vi "Replace Array Elements - string.vi"(4 "new elements (none)":string[](array[string])=["a"], 5 "indices (none)":i32[](array[numeric])=[3, 5], 7 "1D Array":string[](array[string])=["0", "1", "2", "empty", "4", "none", "6", "7", "8"]) -> (2 "output array":string[](array[string]))   [LabVIEW 2020]
doc: "Replaces elements in a 1-dim array at the specified indices. This is a list-based version of the built-in \"Replace Array Subset\"."
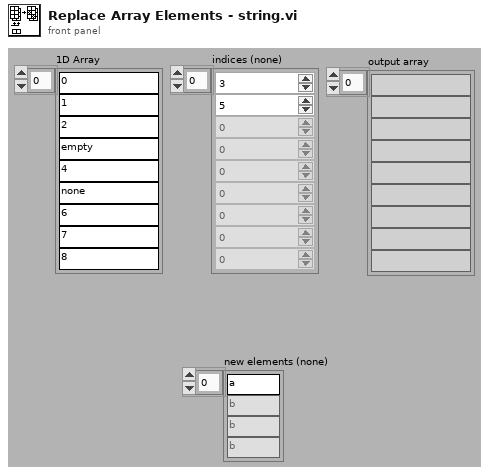
[diagram p1: front panel]
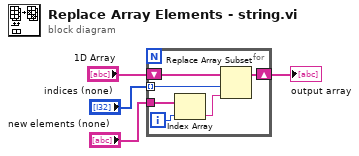
[diagram p0: block diagram]
diagram:
  n1 = for {
    tunnel: "new elements (none)" -> [w8]
    shift-right: [w9] -> w3
    shift-left: "1D Array" -> [w10]
    tunnel: "indices (none)" -> [w6] mode=indexing
    i -> [w5]
    n2 = Index Array(array=w8, index=w5) -> (element=w7:string)
    n3 = Replace Array Subset(array=w10, new element=w7, index=w6) -> (w9:string[])
  }
  "output array" <- w3
